vi "DataTranslation_NM3.vi"() -> ()   [LabVIEW 2011]
doc: "This vi will take data with multiple DT boxes for an arbitrary number of channels either differentially or single ended, depending upon how you have wired the boxes up."
uses:
  Controls/DT_Cluster.ctl
  Controls/DT_Mode.ctl
  Globals/Meas_global.vi
  <userlib>/LV-Link3/PolySubVIs/DtCreateAinChan.vi
  <userlib>/LV-Link3/PolySubVIs/DtCreateCtrRateChan.vi
  <userlib>/LV-Link3/PolySubVIs/DtOLTimingSetInput.vi
  <userlib>/LV-Link3/PolySubVIs/DtOLStartNormal.vi
  <userlib>/LV-Link3/PolySubVIs/DtOLReadMultiple2D.vi
  <userlib>/LV-Link3/PolySubVIs/DtOLTriggerDigital.vi
panel:
  out "DAQ Error":errorcluster
  out "Array":T1[](array[typedef])
  out "Waveform Graph":dbl[][](graph)
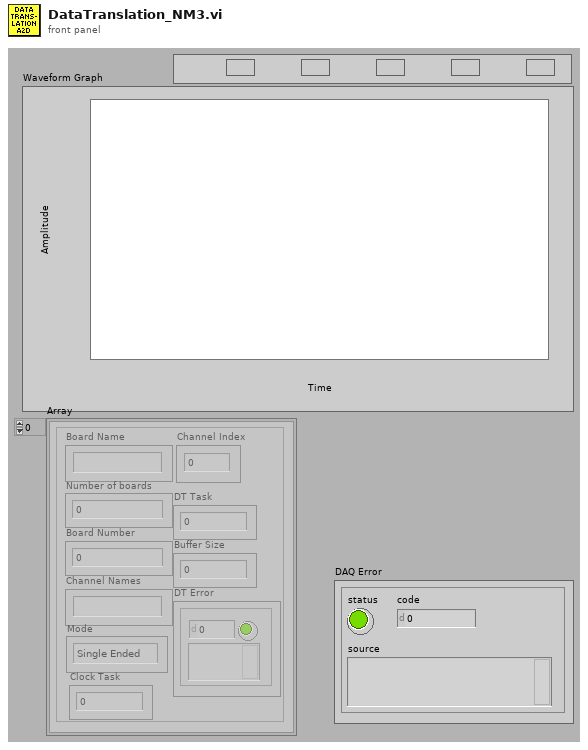
[diagram p1: front panel]
types:
  T1 = typedef "DT_Cluster.ctl" = cluster{"Board Name":string, "Number of boards":u32, "Board Number":u32, "Channel Names":string, "Channel Index":i32[], "DT Task":i32, "DT Error":errorcluster, "Mode":T2, "Buffer Size":u32, "Clock Task":i32}
  T2 = typedef "DT_Mode.ctl" = enum16{"Single Ended", "Differential"}
  T3 = typedef "Trigger_Mode.ctl" = enum16{"Free Running", "Start on Trigger", "Trigger Every Block", "Trigger Every Sample"}
  T4 = enum32{"Invalid", "Standard", "Closed", "Hidden", "Minimized", "Maximized"}
  T5 = enum32{"Internal Clock", "External Clock", "No Timing"}
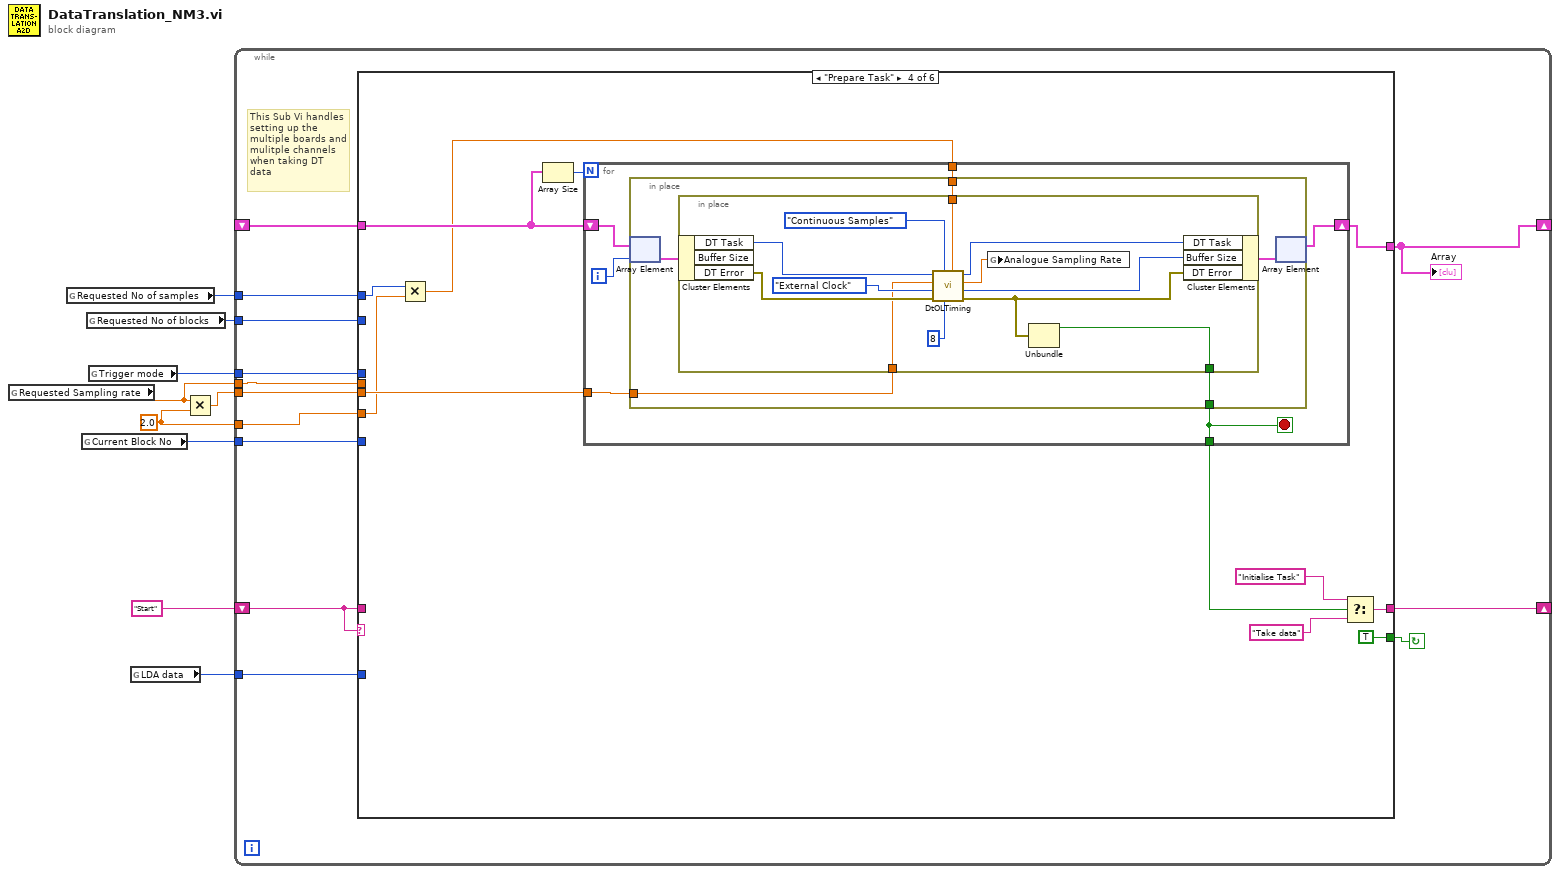
[diagram p0: block diagram]
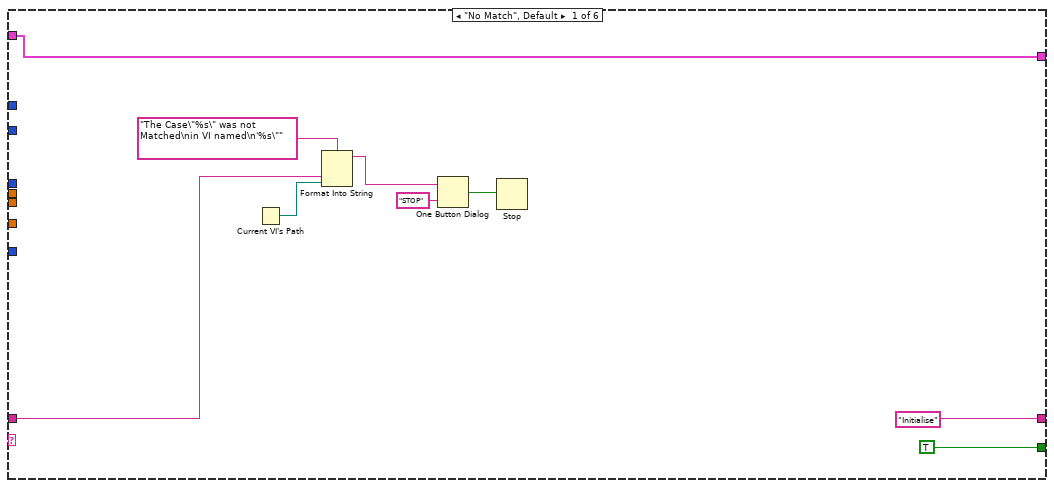
[diagram p2: hidden frame]
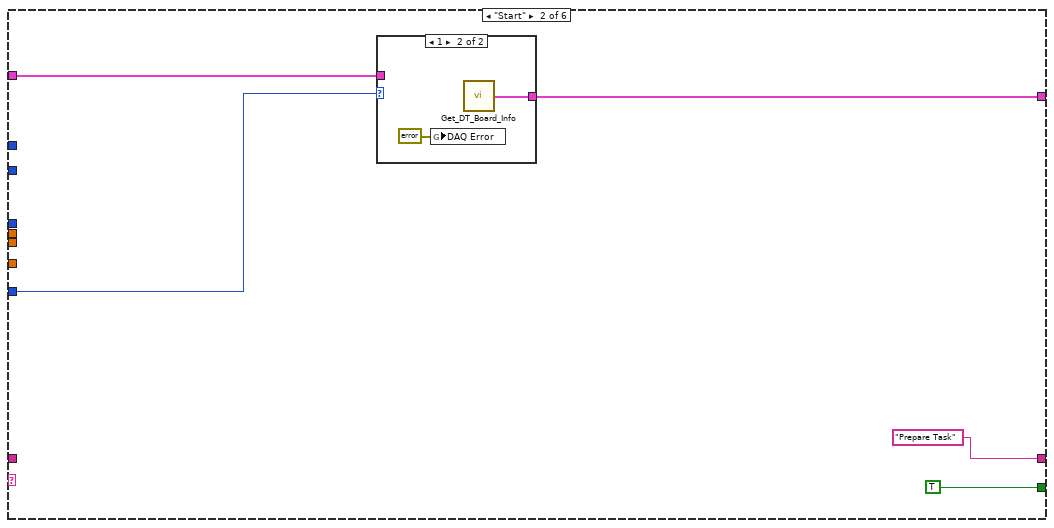
[diagram p3: hidden frame]
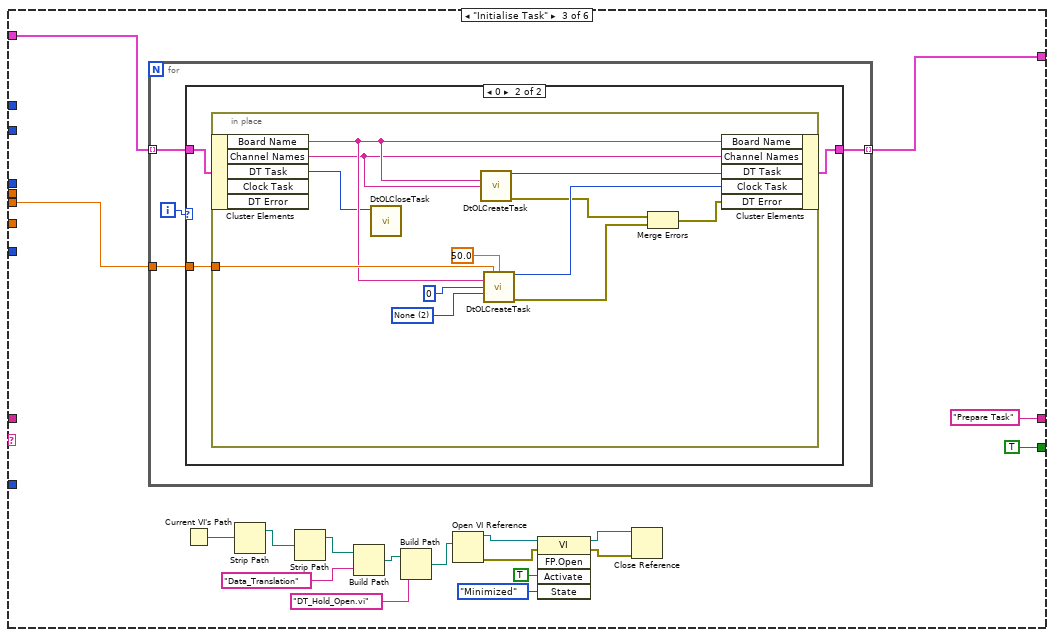
[diagram p5: hidden frame]
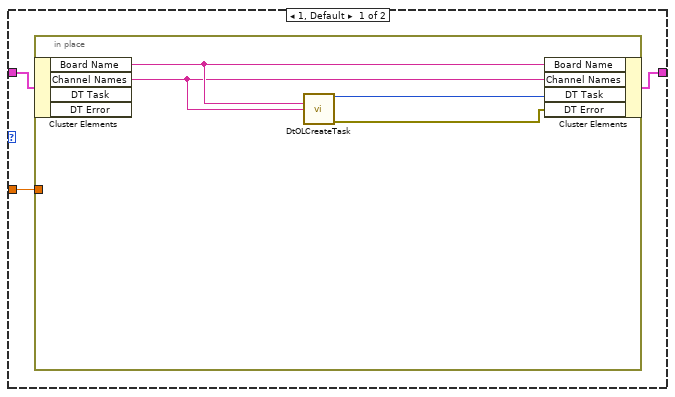
[diagram p6: hidden frame]
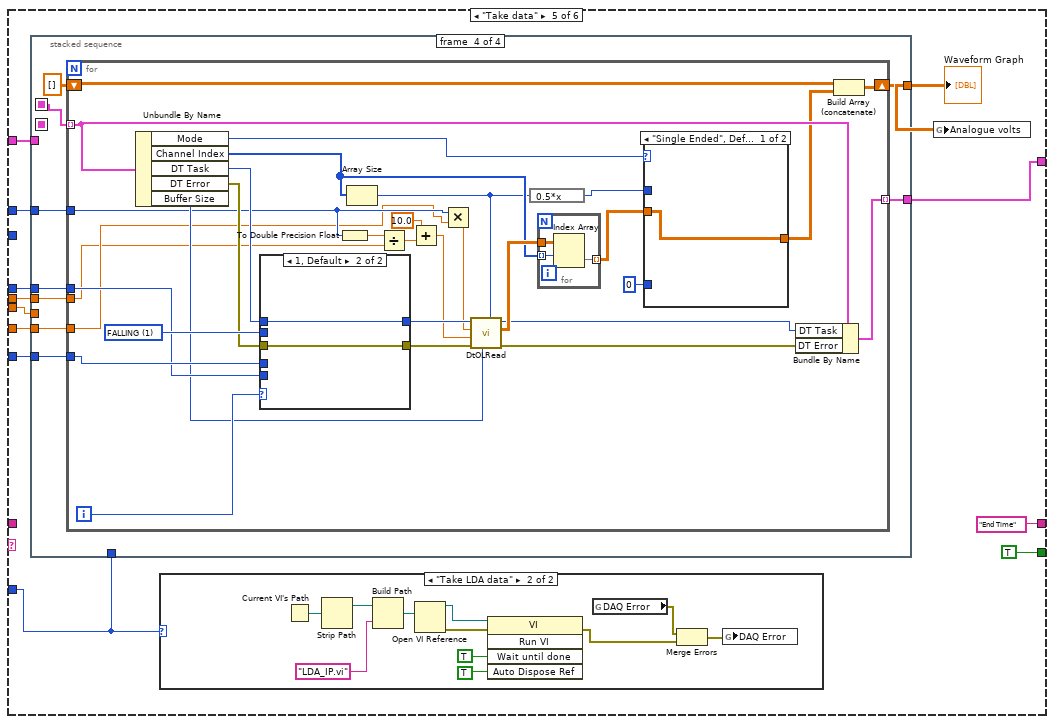
[diagram p7: hidden frame]
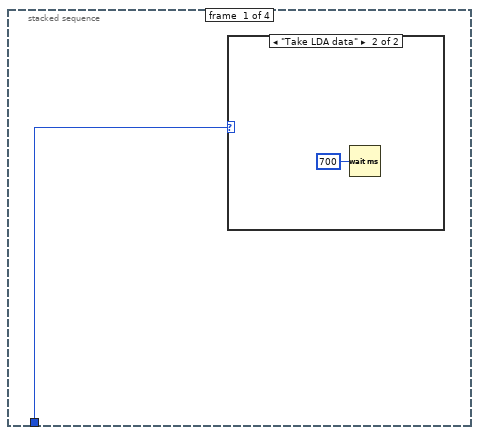
[diagram p9: hidden frame]
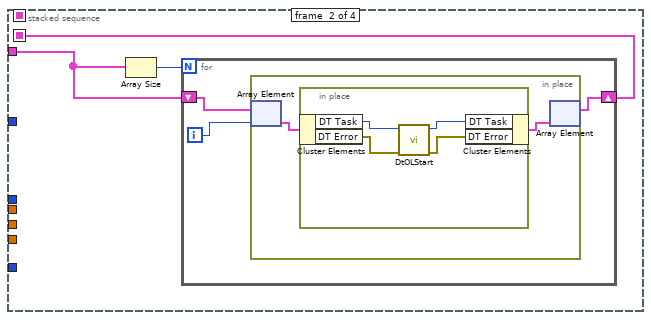
[diagram p11: hidden frame]
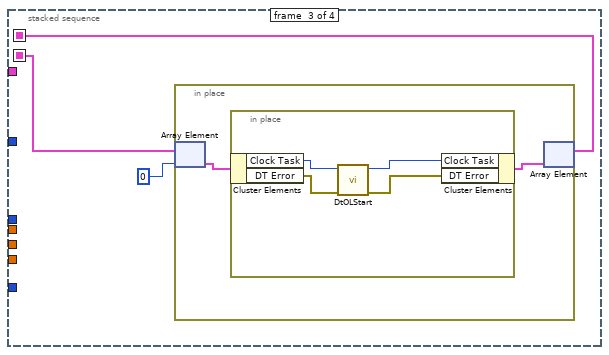
[diagram p12: hidden frame]
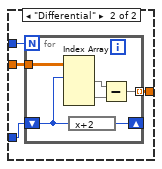
[diagram p13: hidden frame]
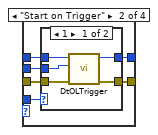
[diagram p16: hidden frame]
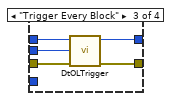
[diagram p18: hidden frame]
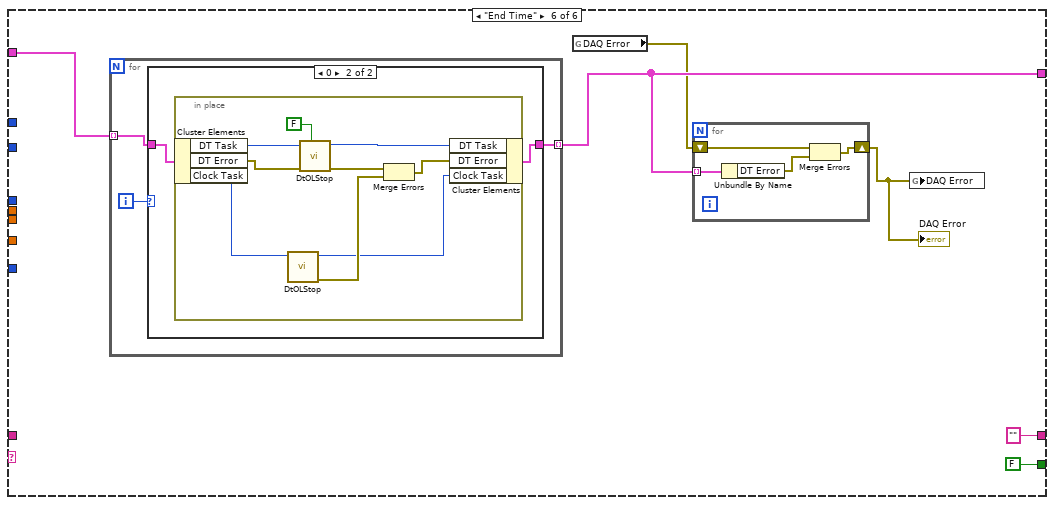
[diagram p19: hidden frame]
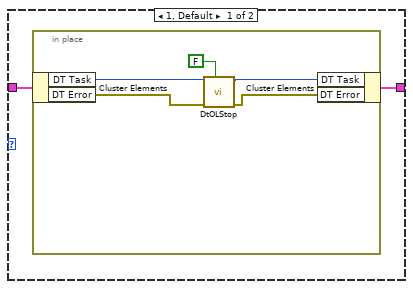
[diagram p20: hidden frame]
diagram:
  w2 = 2.0 ("y")
  n1 = global read "Meas_global.vi" "Requested Sampling rate"() -> (w1:dbl)
  n2 = global read "Meas_global.vi" "Requested No of samples"() -> (w8:i32)
  n3 = global read "Meas_global.vi" "Current Block No"() -> (w6:i32)
  n4 = global read "Meas_global.vi" "Requested No of blocks"() -> (w5:i32)
  n5 = global read "Meas_global.vi" "Trigger mode"() -> (w7:T3)
  n6 = global read "Meas_global.vi" "LDA data"() -> (w4:enum16{"No LDA data", "Take LDA data"})
  n7 = Multiply(x=w1, y=w2) -> (x*y=w3:dbl)
  n8 = while {
    shift-left: "Start" -> [w21]
    shift-right: [w22] -> _
    tunnel: w3 -> [w20]
    tunnel: w8 -> [w19]
    tunnel: w6 -> [w18]
    tunnel: w7 -> [w16]
    tunnel: w5 -> [w15]
    shift-right: [w14] -> _
    shift-left: _ -> [w13]
    tunnel: w4 -> [w12]
    tunnel: w2 -> [w11]
    tunnel: w1 -> [w10]
    stop <- w17 continue-if-true
    # "This Sub Vi handles setting up the multiple boards and mulitple channels when taking DT data"
    n9 = case shown="\"Prepare Task\"" w21 {
      tunnel: ["Initialise" "Prepare Task" "Prepare Task" w92 "End Time" "" ("f")] -> w22
      tunnel: w21 -> [w27 _ _ _ _ _]
      tunnel: w20 -> [_ _ w55 w88 w119 _]
      tunnel: w19 -> [_ _ _ w86 w129 _]
      tunnel: w18 -> [_ w32 _ _ w127 _]
      tunnel: [TRUE TRUE TRUE TRUE TRUE FALSE] -> w17
      tunnel: w16 -> [_ _ _ _ w126 _]
      tunnel: w15 -> [_ _ _ _ _ _]
      tunnel: w13 -> [w23 w34 w40 w87 w125 w253]
      tunnel: [w23 w35 w54 w89 w124 w252] -> w14
      tunnel: w12 -> [_ _ _ _ w120 _]
      tunnel: w11 -> [_ _ _ w85 w122 _]
      tunnel: w10 -> [_ _ _ _ w121 _]
      frame "No Match", Default {
        n10 = Current VI's Path() -> (path=w26:path)
        n11 = Format Into String(format string="The Case\"%s\" was not Matched\nin VI named\n'%s\"" ("Format String"), w27, w26) -> (resulting string=w30:string)  [unwired: 2 in, 1 out]
        n12 = One Button Dialog(message=w30, button name ("OK")="STOP") -> (true=w28:bool)
        n13 = Stop(stop? (T)=w28) -> ()
      }
      frame "Start" {
        n14 = case shown="1" w32 {
          tunnel: [w37 w39] -> w35
          tunnel: w34 -> [w37 _]
          frame 2, Default {
          }
          frame 1 {
            n15 = global write "Meas_global.vi" "DAQ Error"(errorcluster {"status"=FALSE, "code"=0, "source"=""} ("DAQ Error")) -> ()
            n16 = call "Get_DT_Board_Info.vi"() -> ("DT Cluster Array"=w39:T1[])  [unwired: 5 in]
          }
        }
      }
      frame "Initialise Task" {
        n17 = for {
          tunnel: w40 -> [w61] mode=indexing
          tunnel: w55 -> [w60]
          tunnel: [w59] -> w54 mode=indexing
          i -> [w58]
          n18 = case shown="0" w58 {
            tunnel: w61 -> [w64 w71]
            tunnel: w60 -> [w63 w70]
            tunnel: [w62 w69] -> w59
            frame 1, Default {
              n19 = in-place {
                in-place-border: w63 -> [_]
                n20 = in-place-cluster #1(w64) -> ("Board Name"=w68:string, "Channel Names"=w65:string)  [unwired: 2 out]
                n21 = call-poly <userlib>:"DtOLCreateTask.vi"("Board Name"=w68, "Channel"=w65) -> ("Task out"=w67:i32, "error out"=w66:errorcluster)  [unwired: 11 in, 1 out]
                n22 = in-place-cluster #1("Board Name"=w68, "Channel Names"=w65, "DT Task"=w67, "DT Error"=w66) -> (w62:T1)
              }
            }
            frame 0 {
              n23 = in-place {
                in-place-border: w70 -> [w80]
                w83 = 2 items=["LowLevel", "HighLevel", "None"] ("Gate Type")
                n24 = in-place-cluster #2(w71) -> ("Board Name"=w78:string, "Channel Names"=w73:string, "DT Task"=w72:i32)  [unwired: 2 out]
                n25 = call <userlib>:"DtOLCloseTask.vi"("Task in"=w72) -> ()  [unwired: 10 in, 1 out]
                n26 = call-poly <userlib>:"DtOLCreateTask.vi"("Board Name"=w78, "Channel"=w73) -> ("Task out"=w77:i32, "error out"=w75:errorcluster)  [unwired: 11 in, 1 out]
                n27 = call-poly <userlib>:"DtOLCreateTask.vi"("Requested\nFrequency (Hz)"=w80, "Duty Cycle"=50.0, "Board Name"=w78, "Counter Num"=u32 0, "Gate Type"=w83) -> ("Task out"=w76:i32, "error out"=w79:errorcluster)  [unwired: 8 in, 1 out]
                n28 = Merge Errors(w75, w79) -> (w74:errorcluster)
                n29 = in-place-cluster #2("Board Name"=w78, "Channel Names"=w73, "DT Task"=w77, "Clock Task"=w76, "DT Error"=w74) -> (w69:T1)
              }
            }
          }
        }
        n30 = Current VI's Path() -> (path=w53:path)
        n31 = Strip Path(path=w53) -> (stripped path=w52:path)  [unwired: 1 out]
        n32 = Strip Path(path=w52) -> (stripped path=w45:path)  [unwired: 1 out]
        n33 = Build Path(base path=w45, name or relative path="Data_Translation") -> (appended path=w43:path)
        n34 = Build Path(base path=w43, name or relative path="DT_Hold_Open.vi") -> (appended path=w41:path)
        n35 = Open VI Reference(vi path=w41) -> (vi reference=w51:refnum<vi>, error out=w48:errorcluster)  [unwired: 5 in]
        n36 = invoke class="VI" method="FP.Open"(reference=w51, error in=w48, "Activate"=TRUE ("Activate?"), "State"=T4."Minimized") -> (reference out=w47:refnum<vi>, error out=w46:errorcluster)  [unwired: 1 in, 3 out]
        n37 = Close Reference(reference=w47, error in (no error)=w46) -> ()  [unwired: 1 out]
      }
      frame "Prepare Task" {
        n38 = Multiply(x=w86, y=w85) -> (x*y=w84:dbl)
        n39 = Array Size(array=w87) -> (size(s)=w91:i32)
        n40 = for {
          N: w91 -> [_]
          shift-right: [w98] -> w89
          shift-left: w87 -> [w100]
          tunnel: [w101] -> w90
          tunnel: w88 -> [w97]
          tunnel: w84 -> [w96]
          i -> [w99]
          stop <- w101 stop-if-true
          n41 = in-place {
            in-place-border: [w106] -> w101
            in-place-border: w97 -> [w103]
            in-place-border: w96 -> [w102]
            n42 = in-place-array #3(w100, w99) -> (w105:T1)
            n43 = in-place {
              in-place-border: [w109] -> w106
              in-place-border: w103 -> [w108]
              in-place-border: w102 -> [w107]
              n44 = in-place-cluster #4(w105) -> ("DT Task"=w115:i32, "DT Error"=w114:errorcluster)  [unwired: 1 out]
              n45 = call-poly <userlib>:"DtOLTiming.vi"("Samples Per Channel"=w107, "Num Buffers"=u32 8, "Sample Mode"=enum16{"Finite Samples", "Continuous Samples"}."Continuous Samples", "error in (no error)"=w114, "Timing"=T5."External Clock", "Sample Freq (Hz)"=w108, "Task in"=w115) -> ("error out"=w110:errorcluster, "Buffer Size"=w113:u32, "Actual Sample Freq"=w116:dbl, "Task out"=w112:i32)  [unwired: 1 in]
              n46 = global write "Meas_global.vi" "Analogue Sampling Rate"(w116) -> ()
              n47 = Unbundle(w110) -> ("status"=w109:bool)  [unwired: 2 out]
              n48 = in-place-cluster #4("DT Task"=w112, "Buffer Size"=w113, "DT Error"=w110) -> (w104:T1)
            }
            n49 = in-place-array #3(w104) -> (w98:T1[])  [unwired: 1 out]
          }
        }
        n50 = Select(t="Initialise Task", s=w90, f="Take data") -> (s? t:f=w92:string)
      }
      frame "Take data" {
        n51 = stacked-sequence {
          seq-local: [_ w146 _ _] -> [_ _ w157 _]
          seq-local: [_ _ w156 _] -> [_ _ _ w165]
          tunnel: w129 -> [_ _ _ w173]
          tunnel: w127 -> [_ _ _ w172]
          tunnel: w126 -> [_ _ _ w171]
          tunnel: w125 -> [_ w145 _ _]
          tunnel: [_ _ _ w170] -> w124
          tunnel: [_ _ _ w168] -> w123
          tunnel: w122 -> [_ _ _ w167]
          tunnel: w121 -> [_ _ _ w166]
          tunnel: w120 -> [w142 _ _ _]
          tunnel: w119 -> [_ _ _ _]
          frame #0 {
            n52 = case shown="\"Take LDA data\"" w142 {
              frame "No LDA data", Default {
              }
              frame "Take LDA data" {
                n53 = Wait (ms)(milliseconds to wait=u32 700) -> ()  [unwired: 1 out]
              }
            }
          }
          frame #1 {
            n54 = Array Size(array=w145) -> (size(s)=w144:i32)
            n55 = for {
              N: w144 -> [_]
              shift-right: [w147] -> w146
              shift-left: w145 -> [w148]
              i -> [w149]
              n56 = in-place {
                n57 = in-place-array #5(w148, w149) -> (w151:T1)
                n58 = in-place {
                  n59 = in-place-cluster #6(w151) -> ("DT Task"=w155:i32, "DT Error"=w154:errorcluster)
                  n60 = call-poly <userlib>:"DtOLStart.vi"("error in (no error)"=w154, "Task in"=w155) -> ("error out"=w153:errorcluster, "Task out"=w152:i32)  [unwired: 8 in]
                  n61 = in-place-cluster #6("DT Task"=w152, "DT Error"=w153) -> (w150:T1)
                }
                n62 = in-place-array #5(w150) -> (w147:T1[])  [unwired: 1 out]
              }
            }
          }
          frame #2 {
            n63 = in-place {
              n64 = in-place-array #7(w157, 0) -> (w160:T1)
              n65 = in-place {
                n66 = in-place-cluster #8(w160) -> ("Clock Task"=w163:i32, "DT Error"=w164:errorcluster)
                n67 = call-poly <userlib>:"DtOLStart.vi"("error in (no error)"=w164, "Task in"=w163) -> ("error out"=w161:errorcluster, "Task out"=w162:i32)  [unwired: 8 in]
                n68 = in-place-cluster #8("Clock Task"=w162, "DT Error"=w161) -> (w159:T1)
              }
              n69 = in-place-array #7(w159) -> (w156:T1[])  [unwired: 1 out]
            }
          }
          frame #3 {
            n70 = for {
              tunnel: w173 -> [w178]
              tunnel: w172 -> [w202]
              tunnel: w171 -> [w201]
              tunnel: w165 -> [w197] mode=indexing
              tunnel: [w196] -> w170 mode=indexing
              shift-right: [w193] -> w168
              shift-left: dbl[][] [] -> [w192]
              tunnel: w167 -> [w177]
              tunnel: w166 -> [w175]
              i -> [w187]
              w203 = 1 items=["RISING", "FALLING"] ("External Trigger Polarity")
              n71 = Unbundle By Name(w197) -> ("Mode"=w184:T2, "Channel Index"=w194:i32[], "DT Task"=w200:i32, "DT Error"=w199:errorcluster, "Buffer Size"=w180:u32)
              n72 = case shown="1, Default" w187 {
                tunnel: [w222 w246] -> w204
                tunnel: w203 -> [w221 _]
                tunnel: w202 -> [w220 _]
                tunnel: w201 -> [w219 _]
                tunnel: w200 -> [w218 w246]
                tunnel: w199 -> [w217 w245]
                tunnel: [w216 w245] -> w198
                frame 0 {
                  n73 = case shown="\"Trigger Every Sample\"" w219 {
                    tunnel: [w224 w228 w240 w244] -> w222
                    tunnel: w218 -> [w224 w229 w242 w244]
                    tunnel: w220 -> [_ w230 _ _]
                    tunnel: w221 -> [_ w227 w241 _]
                    tunnel: w217 -> [w223 w226 w239 w243]
                    tunnel: [w223 w225 w238 w243] -> w216
                    frame "Free Running" {
                    }
                    frame "Start on Trigger" {
                      n74 = case shown="1" w230 {
                        tunnel: w229 -> [w235 w237]
                        tunnel: w226 -> [w234 w236]
                        tunnel: [w232 w237] -> w228
                        tunnel: [w233 w236] -> w225
                        tunnel: w227 -> [w231 _]
                        frame 1 {
                          n75 = call-poly <userlib>:"DtOLTrigger.vi"("error in (no error)"=w234, "External Trigger Polarity"=w231, "Task in"=w235) -> ("error out"=w233:errorcluster, "Task out"=w232:i32)  [unwired: 7 in]
                        }
                        frame 2, Default {
                        }
                      }
                    }
                    frame "Trigger Every Block" {
                      n76 = call-poly <userlib>:"DtOLTrigger.vi"("error in (no error)"=w239, "External Trigger Polarity"=w241, "Task in"=w242) -> ("error out"=w238:errorcluster, "Task out"=w240:i32)  [unwired: 7 in]
                    }
                    frame "Trigger Every Sample" {
                    }
                  }
                }
                frame 1, Default {
                }
              }
              n77 = To Double Precision Float(number=w178) -> (double precision float=w191:dbl)
              n78 = Array Size(array=w194) -> (size(s)=w182:i32)
              n79 = Divide(x=w191, y=w175) -> (x/y=w190:dbl)
              n80 = Add(x=10.0, y=w190) -> (x+y=w188:dbl)
              n81 = Multiply(x=w178, y=w177) -> (x*y=w176:dbl)
              n82 = call-poly <userlib>:"DtOLRead.vi"("Number Chan to Read"=w182, "Buffer size"=w180, "error in (no error)"=w198, "Timeout"=w188, "Samples Per Channel"=w176, "Task in"=w204) -> ("error out"=w179:errorcluster, "2D Data out"=w195:dbl[][], "Task out"=w186:i32)  [unwired: 1 in, 2 out]
              n83 = expression code="0.5*x"(w182) -> (w181:i32)
              n84 = for {
                tunnel: w194 -> [w249] mode=indexing
                tunnel: w195 -> [w248]
                tunnel: [w247] -> w174 mode=indexing
                n85 = Index Array(array=w248, index (row)=w249) -> (element=w247:dbl[])  [unwired: 1 in]
              }
              n86 = case shown="\"Single Ended\", Default" w184 {
                tunnel: w174 -> [w205 w209]
                tunnel: [w205 w208] -> w185
                tunnel: 0 ("size(s)") -> [_ w207]
                tunnel: w181 -> [_ w206]
                frame "Single Ended", Default {
                }
                frame "Differential" {
                  n87 = for {
                    N: w206 -> [_]
                    tunnel: w209 -> [w215]
                    shift-right: [w214] -> _
                    shift-left: w207 -> [w213]
                    tunnel: [w211] -> w208 mode=indexing
                    n88 = Index Array(array=w215, index (row) #1=w213) -> (element #1=w210:dbl[], element #2=w212:dbl[])  [unwired: 3 in]
                    n89 = expression code="x+2"(w213) -> (w214:i32)
                    n90 = Subtract(x=w210, y=w212) -> (x-y=w211:dbl[])
                  }
                }
              }
              n91 = Bundle By Name(cluster=w197, "DT Task"=w186, "DT Error"=w179) -> (w196:T1)
              n92 = Build Array (concatenate)(w192, w185) -> (w193:dbl[][])
            }
          }
        }
        "Waveform Graph" <- w123
        n93 = case shown="\"Take LDA data\"" w120 {
          frame "No LDA data", Default {
          }
          frame "Take LDA data" {
            n94 = Current VI's Path() -> (path=w135:path)
            n95 = Strip Path(path=w135) -> (stripped path=w131:path)  [unwired: 1 out]
            n96 = Build Path(base path=w131, name or relative path="LDA_IP.vi") -> (appended path=w136:path)
            n97 = Open VI Reference(vi path=w136) -> (vi reference=w139:refnum<vi>, error out=w140:errorcluster)  [unwired: 5 in]
            n98 = invoke class="VI" method="Run VI"(reference=w139, error in=w140, "Wait until done"=TRUE ("Wait Until Done"), "Auto Dispose Ref"=TRUE ("Wait until done")) -> (error out=w133:errorcluster)  [unwired: 1 in, 4 out]
            n99 = global read "Meas_global.vi" "DAQ Error"() -> (w134:errorcluster)
            n100 = Merge Errors(w134, w133) -> (w132:errorcluster)
            n101 = global write "Meas_global.vi" "DAQ Error"(w132) -> ()
          }
        }
        n102 = global write "Meas_global.vi" "Analogue volts"(w123) -> ()
      }
      frame "End Time" {
        n103 = for {
          tunnel: w253 -> [w258] mode=indexing
          tunnel: [w257] -> w252 mode=indexing
          i -> [w256]
          n104 = case shown="0" w256 {
            tunnel: w258 -> [w260 w267]
            tunnel: [w259 w266] -> w257
            frame 1, Default {
              n105 = in-place {
                n106 = in-place-cluster #9(w260) -> ("DT Task"=w265:i32, "DT Error"=w264:errorcluster)
                n107 = call <userlib>:"DtOLStop.vi"("Finish Buffer"=FALSE, "error in (no error)"=w264, "Task in"=w265) -> ("error out"=w261:errorcluster, "Task out"=w263:i32)  [unwired: 7 in]
                n108 = in-place-cluster #9("DT Task"=w263, "DT Error"=w261) -> (w259:T1)
              }
            }
            frame 0 {
              n109 = in-place {
                n110 = in-place-cluster #10(w267) -> ("DT Task"=w274:i32, "DT Error"=w273:errorcluster, "Clock Task"=w269:i32)
                n111 = call <userlib>:"DtOLStop.vi"("Task in"=w269) -> ("error out"=w276:errorcluster, "Task out"=w268:i32)  [unwired: 9 in]
                n112 = call <userlib>:"DtOLStop.vi"("Finish Buffer"=FALSE, "error in (no error)"=w273, "Task in"=w274) -> ("error out"=w272:errorcluster, "Task out"=w271:i32)  [unwired: 7 in]
                n113 = Merge Errors(w272, w276) -> (w275:errorcluster)
                n114 = in-place-cluster #10("DT Task"=w271, "DT Error"=w275, "Clock Task"=w268) -> (w266:T1)
              }
            }
          }
        }
        n115 = global read "Meas_global.vi" "DAQ Error"() -> (w251:errorcluster)
        n116 = for {
          tunnel: w252 -> [w280] mode=indexing
          shift-right: [w277] -> w250
          shift-left: w251 -> [w278]
          n117 = Unbundle By Name(w280) -> ("DT Error"=w279:errorcluster)
          n118 = Merge Errors(w278, w279) -> (w277:errorcluster)
        }
        "DAQ Error" <- w250
        n119 = global write "Meas_global.vi" "DAQ Error"(w250) -> ()
      }
    }
    "Array" <- w14
  }
